vi "fg_constants.vi"() -> (1 "table out":string, 2 "schema out":string)   [LabVIEW 2015, in "lv-example-postgres.lvlib"]
uses:
  lv-example-postgres.lvlib
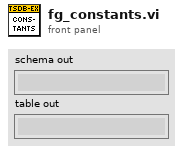
[diagram p1: front panel]
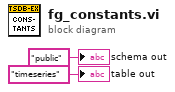
[diagram p0: block diagram]
diagram:
  "table out" <- "timeseries" ("table out")
  "schema out" <- "public" ("schema out")
